vi "Gestione filtri.vi"() -> ()   [LabVIEW 2019]
uses:
  TypeDef/MISURE NM.ctl
  TypeDef/Collegamenti_elettrici.ctl
  TypeDef/Control Calcoli.ctl
  Global percorso impostazioni.vi
  <vilib>/Utility/file.llb/Write Delimited Spreadsheet (string).vi
  <vilib>/Utility/file.llb/Read Delimited Spreadsheet (string).vi
panel:
  in  "REINIZIALIZZA NOMI RIGHE":bool
  in  "Salva FILTRI":bool
  in  "REINIZIALIZZA TABELLA FILTRI":bool
  in  "Salva tipi di collegamento":bool
  in  "EXIT":bool
  in  "ELIMINA TIPO COLLEGAMENTO":bool
  in  "INSERISCI TIPO COLLEGAMENTO":bool
  in  "TIPO COLLEGAMENTO":T3
  in  "DEFINIZIONI TIPI DI COLLEGAMENTO":i32(listbox)
  in  "MISURE NM":T4
  in  "TABELLA FILTRI":string[][](table)
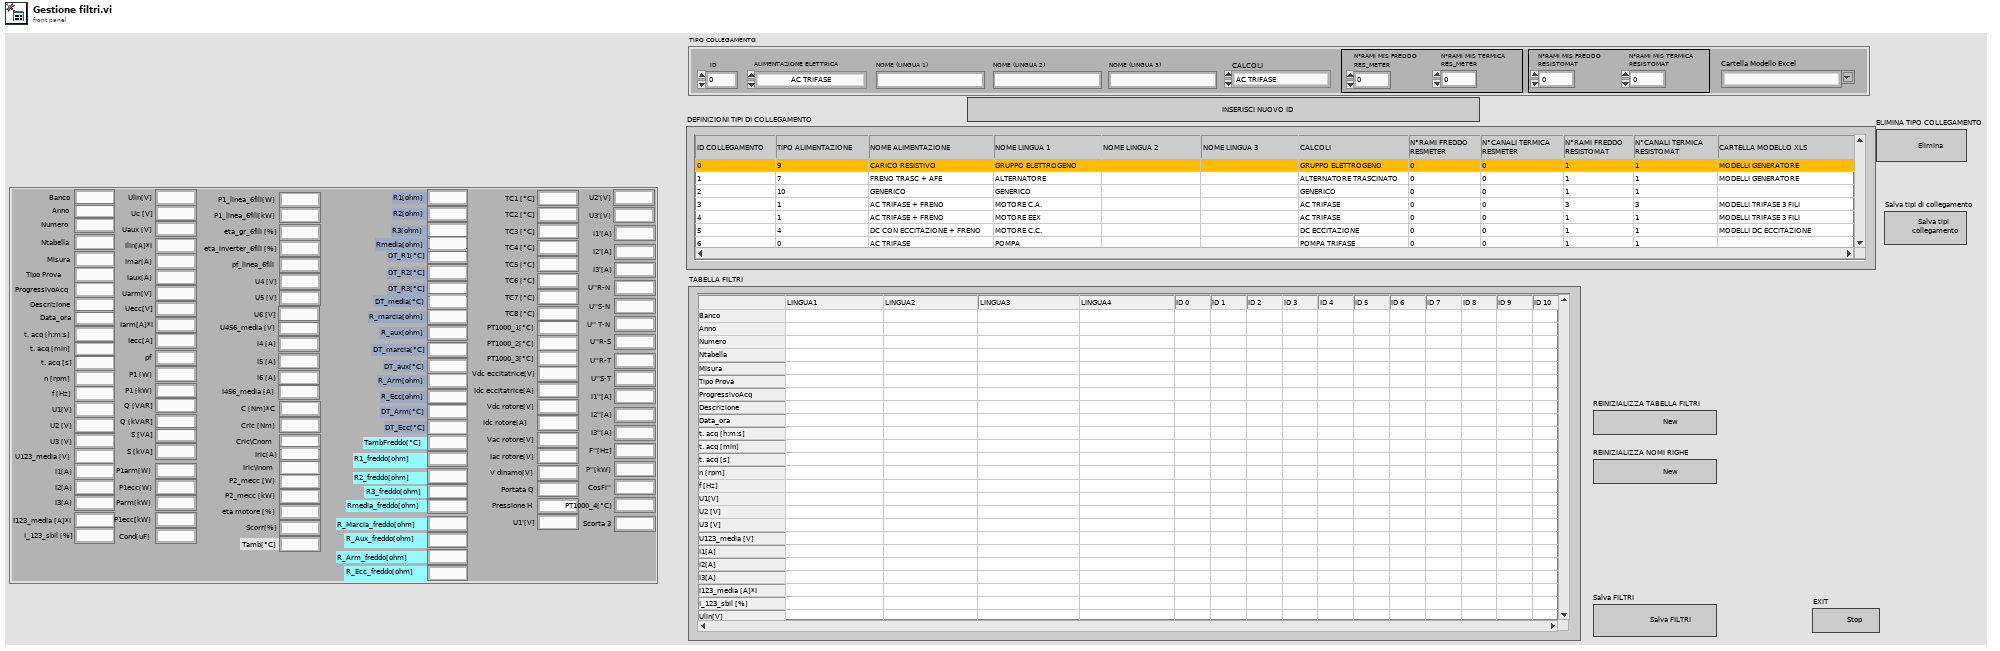
[diagram p1: front panel]
types:
  T1 = typedef "Collegamenti_elettrici.ctl" = enum16{"AC TRIFASE", "AC TRIFASE + FRENO", "AC MONOFASE", "DC CON ECCITAZIONE", "DC CON ECCITAZIONE + FRENO", "DC NO ECCITAZIONE", "DC NO ECCITAZIONE + FRENO", "FRENO TRASC + AFE", "SOLO FRENO", "CARICO RESISTIVO", "GENERICO", "SOLO ACQUISITORE", "SCORTA 4", "SCORTA 5", "SCORTA 6"}
  T2 = typedef "Control Calcoli.ctl" = enum16{"AC TRIFASE", "AC MONOFASE", "DC ECCITAZIONE", "DC NO ECCITAZIONE", "POMPA TRIFASE", "POMPA MONOFASE", "GENERICO", "TRASFORMATORE", "ALTERNATORE TRASCINATO", "GRUPPO ELETTROGENO"}
  T3 = cluster{"IDENTIFICATIVO":i16, "ALIMENTAZIONE ELETTRICA":T1, "NOME (LINGUA 1)":string, "NOME (LINGUA 2)":string, "NOME (LINGUA 3)":string, "N°RAMI MIS FREDDO RES_METER":i16, "N°RAMI MIS TERMICA RES_METER":i16, "N°RAMI MIS FREDDO RESISTOMAT":i16, "N°RAMI MIS TERMICA RESISTOMAT":i16, "Cartella Modello Excel":string, "CALCOLI":T2}
  T4 = typedef "MISURE NM.ctl" = cluster{"Banco":string, "Anno":string, "Numero":string, "Ntabella":string, "Misura":string, "Tipo Prova":string, "ProgressivoAcq":string, "Descrizione":string, "Data_ora":string, "t. acq [h:m:s]":string, "t. acq [min]":string, "t. acq [s]":string, "n [rpm]":string, "f [Hz]":string, "U1[V]":string, "U2 [V]":string, "U3 [V]":string, "U123_media [V]":string, "I1[A]":string, "I2[A]":string, "I3[A]":string, "I123_media [A]*I":string, "I_123_sbil [%]":string, "Ulin[V]":string, "Uc [V]":string, "Uaux [V]":string, "Ilin[A]*I":string, "Imar[A]":string, "Iaux[A]":string, "Uarm[V]":string, "Uecc[V]":string, "Iarm[A]*I":string, "Iecc[A]":string, "pf":string, "P1 [W]":string, "P1 [kW]":string, "Q [VAR]":string, "Q [kVAR]":string, "S [VA]":string, "S [kVA]":string, "P1arm[W]":string, "P1ecc[W]":string, "Parm[kW]":string, "P1ecc[kW]":string, "Cond[uF]":string, "P1_linea_6fili[W]":string, "P1_linea_6fili[kW]":string, "eta_gr_6fili [%]":string, "eta_inverter_6fili [%]":string, "pf_linea_6fili":string, "U4 [V]":string, "U5 [V]":string, "U6 [V]":string, "U456_media [V]":string, "I4 [A]":string, "I5 [A]":string, "I6 [A]":string, "I456_media [A]":string, "C [Nm]*C":string, "Cric [Nm]":string, "Cric\\Cnom":string, "Iric[A]":string, "Iric\\Inom":string, "P2_mecc [W]":string, "P2_mecc [kW]":string, "eta motore [%]":string, "Scorr[%]":string, "Tamb[°C]":string, "R1[ohm]":string, "R2[ohm]":string, "R3[ohm]":string, "Rmedia[ohm]":string, "DT_R1[°C]":string, "DT_R2[°C]":string, "DT_R3[°C]":string, "DT_media[°C]":string, "R_marcia[ohm]":string, "R_aux[ohm]":string, "DT_marcia[°C]":string, "DT_aux[°C]":string, "R_Arm[ohm]":string, "R_Ecc[ohm]":string, "DT_Arm[°C]":string, "DT_Ecc[°C]":string, "TambFreddo[°C]":string, "R1_freddo[ohm]":string, "R2_freddo[ohm]":string, "R3_freddo[ohm]":string, "Rmedia_freddo[ohm]":string, "R_Marcia_freddo[ohm]":string, "R_Aux_freddo[ohm]":string, "R_Arm_freddo[ohm]":string, "R_Ecc_freddo[ohm]":string, "TC1 [°C]":string, "TC2 [°C]":string, "TC3 [°C]":string, "TC4 [°C]":string, "TC5 [°C]":string, "TC6 [°C]":string, "TC7 [°C]":string, "TC8 [°C]":string, "PT1000_1[°C]":string, "PT1000_2[°C]":string, "PT1000_3[°C]":string, "Vdc eccitatrice[V]":string, "Idc eccitatrice[A]":string, "Vdc rotore[V]":string, "Idc rotore[A]":string, "Vac rotore[V]":string, "Iac rotore[V]":string, "V dinamo[V]":string, "Portata Q":string, "Pressione H":string, "U1'[V]":string, "U2'[V]":string, "U3'[V]":string, "I1'[A]":string, "I2'[A]":string, "I3'[A]":string, "U''R-N":string, "U''S-N":string, "U'' T-N":string, "U''R-S":string, "U''R-T":string, "U''S-T":string, "I1''[A]":string, "I2''[A]":string, "I3''[A]":string, "F''[Hz]":string, "P''[kW]":string, "CosFi''":string, "PT1000_4[°C]":string, "Scorta 3":string}
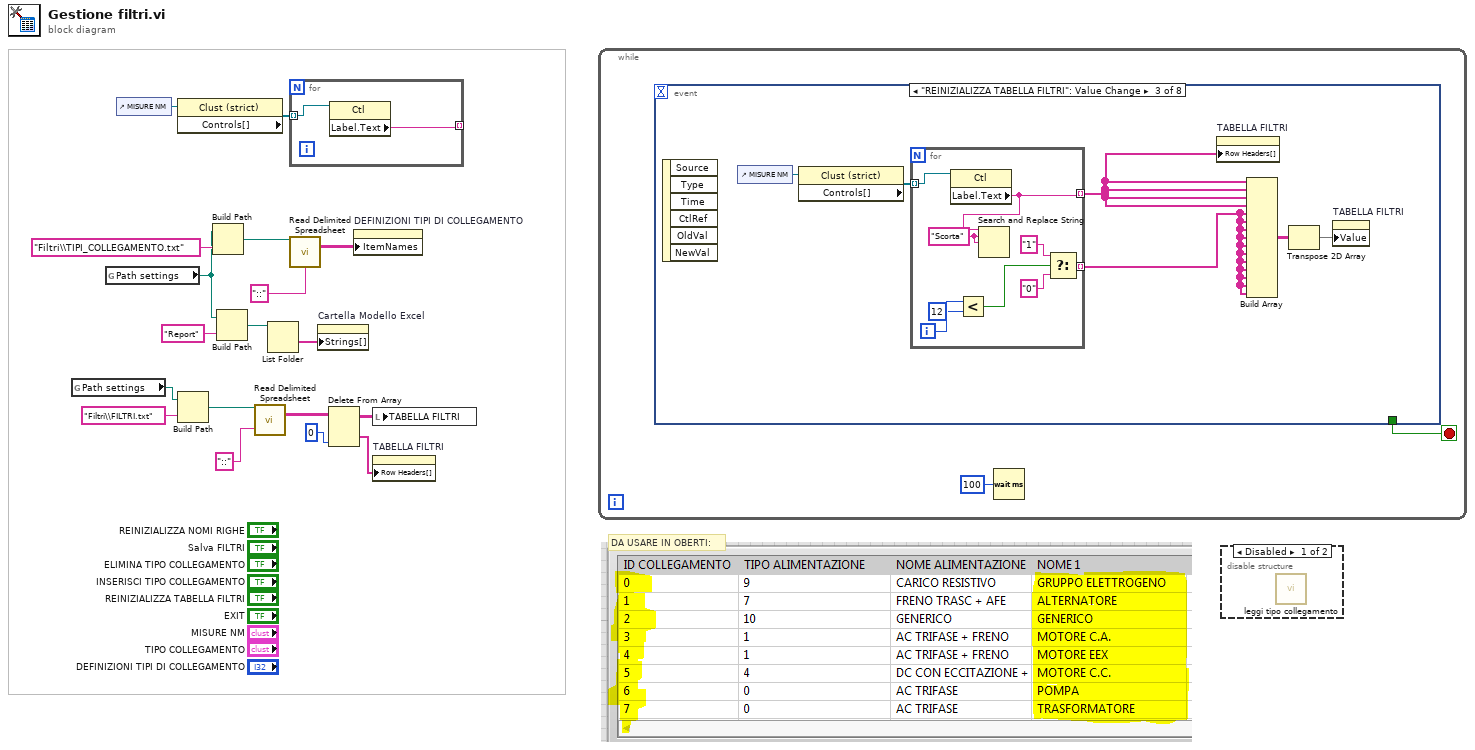
[diagram p0: block diagram]
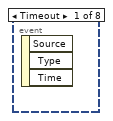
[diagram p3: hidden frame]
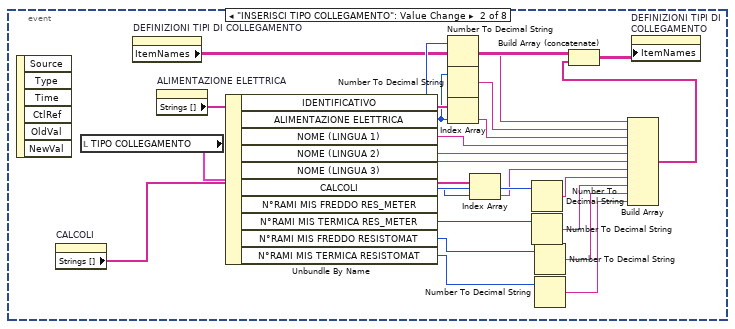
[diagram p4: hidden frame]
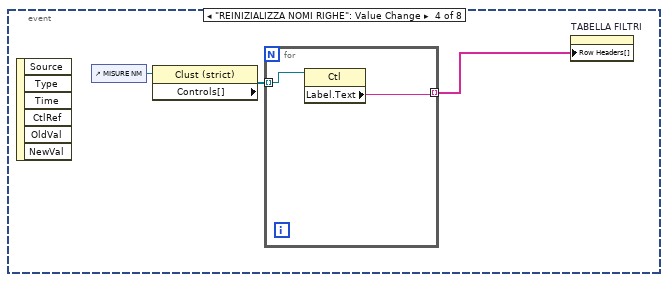
[diagram p5: hidden frame]
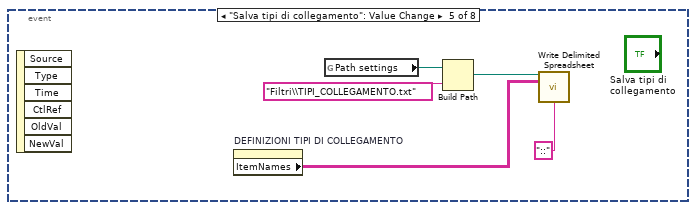
[diagram p6: hidden frame]
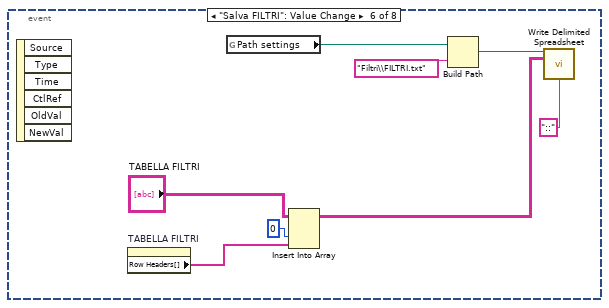
[diagram p7: hidden frame]
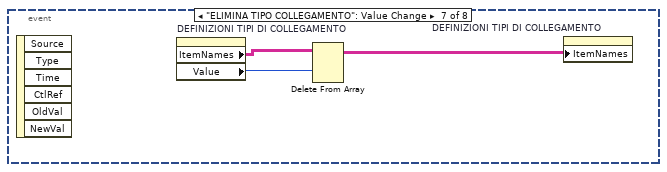
[diagram p8: hidden frame]
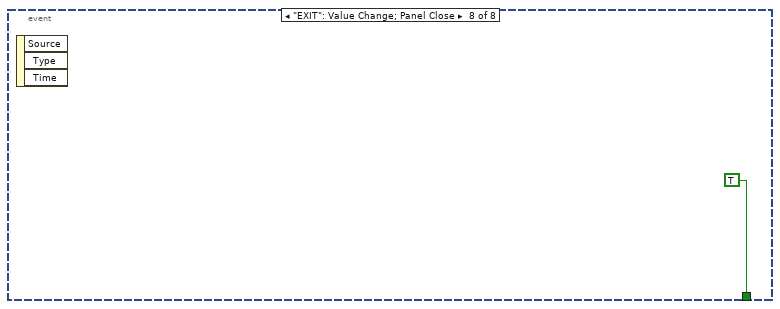
[diagram p9: hidden frame]
diagram:
  # "DA USARE IN OBERTI:"
  n1 = global read "Global percorso impostazioni.vi" "Path settings"() -> (w15:path)
  n2 = global read "Global percorso impostazioni.vi" "Path settings"() -> (w4:path)
  n3 = control-ref of="MISURE NM"() -> (w13:refnum<vi>)
  n4 = property class="Clust (strict)"(reference=w13) -> ("Controls[]"=w12:refnum<vi>[])  [unwired: 1 in, 2 out]
  n5 = Build Path(base path=w15, name or relative path="Filtri\\FILTRI.txt") -> (appended path=w16:path)
  n6 = Build Path(base path=w4, name or relative path="Filtri\\TIPI_COLLEGAMENTO.txt") -> (appended path=w10:path)
  n7 = Build Path(base path=w4, name or relative path="Report") -> (appended path=w2:path)
  n8 = call-poly <vilib>:"Read Delimited Spreadsheet.vi"("file path (dialog if empty)"=w16, "delimiter (\\t)"="::") -> ("all rows"=w18:string[][])  [unwired: 8 in, 5 out]
  n9 = List Folder(path=w2) -> (folder names=w1:string[])  [unwired: 3 in, 3 out]
  n10 = for {
    tunnel: [w20] -> _ mode=indexing
    tunnel: w12 -> [w19] mode=indexing
    n11 = property class="Ctl"(reference=w19) -> ("Label.Text"=w20:string)  [unwired: 1 in, 2 out]
  }
  n12 = call-poly <vilib>:"Read Delimited Spreadsheet.vi"("file path (dialog if empty)"=w10, "delimiter (\\t)"="::") -> ("all rows"=w11:string[][])  [unwired: 8 in, 5 out]
  n13 = property on="Cartella Modello Excel" class="CmbBox"("Strings[]"=w1) -> ()  [unwired: 2 in, 2 out]
  n14 = Delete From Array(array=w18, index (col)=0 ("disabled index (col)")) -> (deleted portion=w5:string[], array with subset deleted=w7:string[][])  [unwired: 2 in]
  n15 = property on="DEFINIZIONI TIPI DI COLLEGAMENTO" class="MCListbox (strict)"("ItemNames"=w11) -> ()  [unwired: 2 in, 2 out]
  n16 = local write "TABELLA FILTRI"(w7) -> ()
  n17 = property on="TABELLA FILTRI" class="Tbl (strict)"("Row Headers[]"=w5) -> ()  [unwired: 2 in, 2 out]
  n18 = while {
    stop <- w22 stop-if-true
    n19 = event shown="[2] \"REINIZIALIZZA TABELLA FILTRI\": Value Change" {
      selector: _ -> [_ _ _ _ _ _ _ _]
      dyn-events: _ -> [_ _ _ _ _ _ _ _]
      timeout: _ -> [_ _ _ _ _ _ _ _]
      tunnel: [_ _ _ _ _ _ _ TRUE] -> w22
      event Timeout {
        n20 = event-data() -> ()  [unwired: 1 in, 3 out]
      }
      event "INSERISCI TIPO COLLEGAMENTO": Value Change {
        n21 = event-data() -> ()  [unwired: 1 in, 6 out]
        n22 = property on="CALCOLI" class="Enum (strict)"() -> ("Strings []"=w24:string[])  [unwired: 2 in, 2 out]
        n23 = local read "TIPO COLLEGAMENTO"() -> (w46:T3)
        n24 = property on="DEFINIZIONI TIPI DI COLLEGAMENTO" class="MCListbox (strict)"() -> ("ItemNames"=w39:string[][])  [unwired: 2 in, 2 out]
        n25 = property on="ALIMENTAZIONE ELETTRICA" class="Enum (strict)"() -> ("Strings []"=w45:string[])  [unwired: 2 in, 2 out]
        n26 = Unbundle By Name(w46) -> ("IDENTIFICATIVO"=w44:i16, "ALIMENTAZIONE ELETTRICA"=w32:T1, "NOME (LINGUA 1)"=w42:string, "NOME (LINGUA 2)"=w41:string, "NOME (LINGUA 3)"=w40:string, "CALCOLI"=w25:T2, "N°RAMI MIS FREDDO RES_METER"=w37:i16, "N°RAMI MIS TERMICA RES_METER"=w35:i16, "N°RAMI MIS FREDDO RESISTOMAT"=w30:i16, "N°RAMI MIS TERMICA RESISTOMAT"=w29:i16)
        n27 = Number To Decimal String(number=w44) -> (decimal integer string=w33:string)  [unwired: 1 in]
        n28 = Number To Decimal String(number=w32) -> (decimal integer string=w31:string)  [unwired: 1 in]
        n29 = Index Array(array=w45, index=w32) -> (element=w43:string)
        n30 = Index Array(array=w24, index=w25) -> (element=w23:string)
        n31 = Number To Decimal String(number=w37) -> (decimal integer string=w36:string)  [unwired: 1 in]
        n32 = Number To Decimal String(number=w35) -> (decimal integer string=w34:string)  [unwired: 1 in]
        n33 = Number To Decimal String(number=w30) -> (decimal integer string=w28:string)  [unwired: 1 in]
        n34 = Number To Decimal String(number=w29) -> (decimal integer string=w27:string)  [unwired: 1 in]
        n35 = Build Array(w33, w31, w43, w42, w41, w40, w23, w36, w34, w28, w27) -> (w26:string[])
        n36 = Build Array (concatenate)(w39, w26) -> (w38:string[][])
        n37 = property on="DEFINIZIONI TIPI DI COLLEGAMENTO" class="MCListbox (strict)"("ItemNames"=w38) -> ()  [unwired: 2 in, 2 out]
      }
      event "REINIZIALIZZA TABELLA FILTRI": Value Change {
        n38 = event-data() -> ()  [unwired: 1 in, 6 out]
        n39 = control-ref of="MISURE NM"() -> (w48:refnum<vi>)
        n40 = property class="Clust (strict)"(reference=w48) -> ("Controls[]"=w49:refnum<vi>[])  [unwired: 1 in, 2 out]
        n41 = for {
          tunnel: [w60] -> w52 mode=indexing
          tunnel: w49 -> [w61] mode=indexing
          tunnel: [w56] -> w47 mode=indexing
          i -> [w55]
          w59 = "Scorta" ("search string")
          n42 = property class="Ctl"(reference=w61) -> ("Label.Text"=w60:string)  [unwired: 1 in, 2 out]
          n43 = Less?(x=w55, y=12) -> (x < y?=w53:bool)
          n44 = Search and Replace String(input string=w60, search string=w59, replace string=w59) -> ()  [unwired: 5 in, 4 out]
          n45 = Select(t="1", s=w53, f="0") -> (s? t:f=w56:string)
        }
        n46 = property on="TABELLA FILTRI" class="Tbl (strict)"("Row Headers[]"=w52) -> ()  [unwired: 2 in, 2 out]
        n47 = Build Array(w52, w52, w52, w52, w47, w47, w47, w47, w47, w47, w47, w47, w47, w47, w47) -> (w50:string[][])
        n48 = Transpose 2D Array(2D array=w50) -> (transposed array=w51:string[][])
        n49 = property on="TABELLA FILTRI" class="Tbl (strict)"("Value"=w51) -> ()  [unwired: 2 in, 2 out]
      }
      event "REINIZIALIZZA NOMI RIGHE": Value Change {
        n50 = event-data() -> ()  [unwired: 1 in, 6 out]
        n51 = control-ref of="MISURE NM"() -> (w62:refnum<vi>)
        n52 = property class="Clust (strict)"(reference=w62) -> ("Controls[]"=w63:refnum<vi>[])  [unwired: 1 in, 2 out]
        n53 = for {
          tunnel: [w65] -> w64 mode=indexing
          tunnel: w63 -> [w66] mode=indexing
          n54 = property class="Ctl"(reference=w66) -> ("Label.Text"=w65:string)  [unwired: 1 in, 2 out]
        }
        n55 = property on="TABELLA FILTRI" class="Tbl (strict)"("Row Headers[]"=w64) -> ()  [unwired: 2 in, 2 out]
      }
      event "Salva tipi di collegamento": Value Change {
        n56 = event-data() -> ()  [unwired: 1 in, 6 out]
        n57 = property on="DEFINIZIONI TIPI DI COLLEGAMENTO" class="MCListbox (strict)"() -> ("ItemNames"=w67:string[][])  [unwired: 2 in, 2 out]
        n58 = global read "Global percorso impostazioni.vi" "Path settings"() -> (w69:path)
        n59 = Build Path(base path=w69, name or relative path="Filtri\\TIPI_COLLEGAMENTO.txt") -> (appended path=w71:path)
        n60 = call-poly <vilib>:"Write Delimited Spreadsheet.vi"("file path (dialog if empty)"=w71, "2D data"=w67, "delimiter (\\t)"="::") -> ()  [unwired: 11 in, 2 out]
      }
      event "Salva FILTRI": Value Change {
        n61 = event-data() -> ()  [unwired: 1 in, 6 out]
        n62 = property on="TABELLA FILTRI" class="Tbl (strict)"() -> ("Row Headers[]"=w73:string[])  [unwired: 2 in, 2 out]
        n63 = global read "Global percorso impostazioni.vi" "Path settings"() -> (w77:path)
        n64 = Insert Into Array "Insert Into Array"(array="TABELLA FILTRI", index (col)=0 ("disabled index (col)"), new element=w73) -> (w72:string[][])  [unwired: 1 in]
        n65 = Build Path(base path=w77, name or relative path="Filtri\\FILTRI.txt") -> (appended path=w79:path)
        n66 = call-poly <vilib>:"Write Delimited Spreadsheet.vi"("file path (dialog if empty)"=w79, "2D data"=w72, "delimiter (\\t)"="::") -> ()  [unwired: 11 in, 2 out]
      }
      event "ELIMINA TIPO COLLEGAMENTO": Value Change {
        n67 = event-data() -> ()  [unwired: 1 in, 6 out]
        n68 = property on="DEFINIZIONI TIPI DI COLLEGAMENTO" class="MCListbox (strict)"() -> ("ItemNames"=w80:string[][], "Value"=w81:i32)  [unwired: 2 in, 2 out]
        n69 = Delete From Array(array=w80, index (row)=w81) -> (array with subset deleted=w82:string[][])  [unwired: 2 in, 1 out]
        n70 = property on="DEFINIZIONI TIPI DI COLLEGAMENTO" class="MCListbox (strict)"("ItemNames"=w82) -> ()  [unwired: 2 in, 2 out]
      }
      event "EXIT": Value Change; Panel Close {
        n71 = event-data() -> ()  [unwired: 1 in, 3 out]
      }
    }
    n72 = Wait (ms)(milliseconds to wait=u32 100) -> ()  [unwired: 1 out]
  }
  n73 = disable-structure shown="Disabled" {
    frame Disabled {
      n74 = call "leggi tipo collegamento.vi"() -> ()  [unwired: 6 in, 6 out]
    }
    frame Enabled {
    }
  }
